vi "LED Main.vi"   [LabVIEW 2016]
uses:
  GlobalVI.vi
  <vilib>/Utility/error.llb/Error Cluster From Error Code.vi
  <vilib>/rvi/errors/niLvFpgaAdjustHostInterfaceError.vi
  <vilib>/rvi/interface/nirviMethod/nirviMethod.xnode
  <vilib>/FPGAPlugInAG/Dynamic/niLvFpga_WriteFifo_Dynamic.vi
  <vilib>/rvi/errors/niLvFpgaMergeErrorWithErrorCode.vi
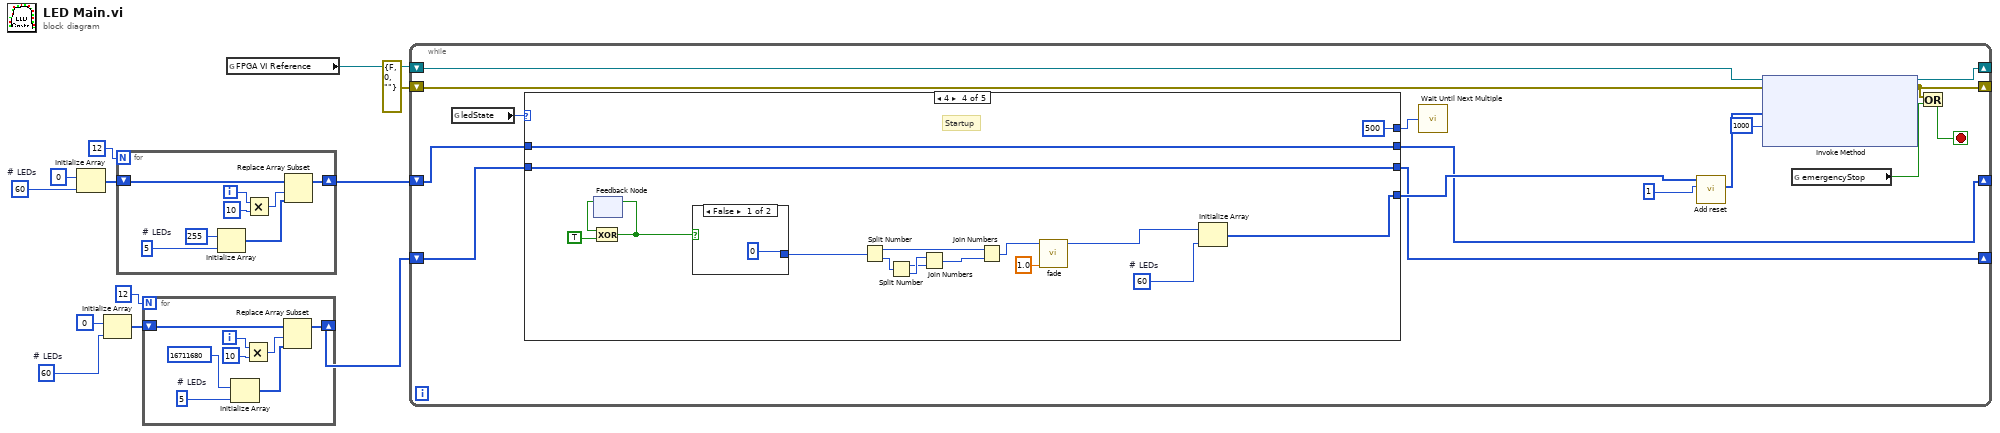
[diagram p0: block diagram]
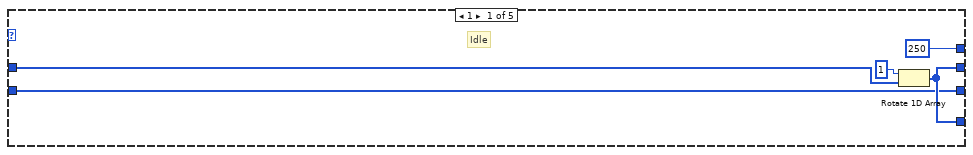
[diagram p2: hidden frame]
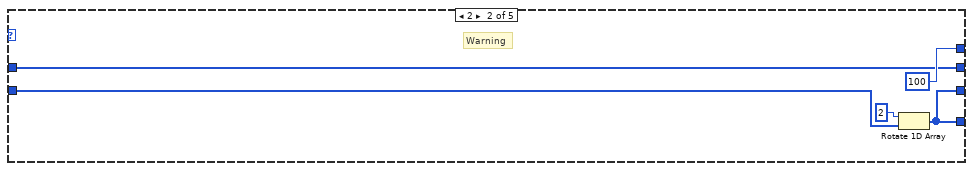
[diagram p3: hidden frame]
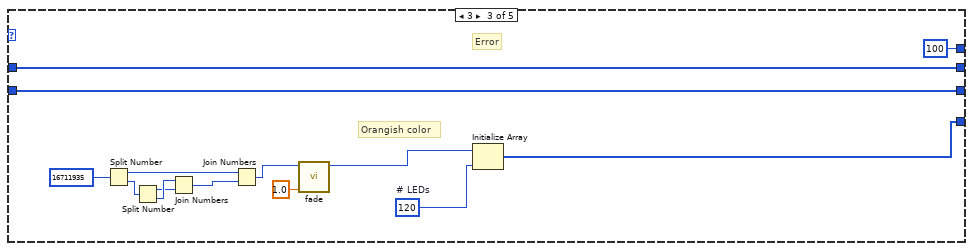
[diagram p4: hidden frame]
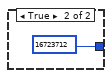
[diagram p5: hidden frame]
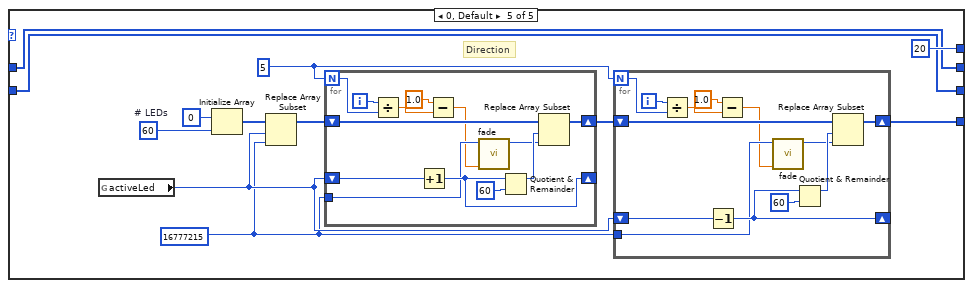
[diagram p6: hidden frame]
diagram:
  w7 = 60  # # LEDs
  w11 = 60  # # LEDs
  n1 = Initialize Array(u32 0 ("Color"), w11) -> (w9:u32[])
  n2 = Initialize Array(u32 0 ("Color"), w7) -> (w5:u32[])
  n3 = for {
    N: 12 -> [_]
    shift-right: [w19] -> w4
    shift-left: w9 -> [w20]
    i -> [w15]
    w18 = 5  # # LEDs
    n4 = Initialize Array(u32 255 ("Color"), w18) -> (w16:u32[])
    n5 = Multiply(x=w15, y=10) -> (x*y=w13:i32)
    n6 = Replace Array Subset(array=w20, new element=w16, index=w13) -> (w19:u32[])
  }
  n7 = for {
    N: 12 -> [_]
    shift-right: [w27] -> w3
    shift-left: w5 -> [w28]
    i -> [w23]
    w26 = 5  # # LEDs
    n8 = Initialize Array(u32 16711680 ("Color"), w26) -> (w24:u32[])
    n9 = Multiply(x=w23, y=10) -> (x*y=w21:i32)
    n10 = Replace Array Subset(array=w28, new element=w24, index=w21) -> (w27:u32[])
  }
  n11 = global read "GlobalVI.vi" "FPGA VI Reference"() -> (w2:refnum<k20>)
  n12 = while {
    shift-right: [w41] -> _
    shift-left: errorcluster {"status"=FALSE, "code"=0, "source"=""} ("error out") -> [w29]
    shift-right: [w44] -> _
    shift-left: w2 -> [w43]
    shift-right: [w32] -> _
    shift-left: w3 -> [w35]
    shift-right: [w33] -> _
    shift-left: w4 -> [w34]
    stop <- w40 stop-if-true
    n13 = global read "GlobalVI.vi" "ledState"() -> (w31:i32)
    n14 = case shown="4" w31 {
      tunnel: [w46 w50 w64 w73 w94] -> w37
      tunnel: [u32 250 ("Count(mSec)") u32 100 ("Count(mSec)") u32 100 ("Count(mSec)") u32 500 ("Count(mSec)") u32 20 ("Count(mSec)")] -> w36
      tunnel: w34 -> [w47 w51 w68 w75 w91]
      tunnel: w35 -> [w45 w52 w65 w74 w92]
      tunnel: [w46 w51 w68 w75 w91] -> w33
      tunnel: [w45 w50 w65 w74 w92] -> w32
      frame 1 {
        # "Idle"
        n15 = Rotate 1D Array(1:w47, 2:1 ("n")) -> (0:w46:u32[])
      }
      frame 2 {
        # "Warning"
        n16 = Rotate 1D Array(1:w52, 2:2 ("n")) -> (0:w50:u32[])
      }
      frame 3 {
        w67 = 120  # # LEDs
        # "Error"
        # "Orangish color"
        n17 = Split Number(x=u32 16711935) -> (hi(x)=w59:u16, lo(x)=w63:u16)
        n18 = Split Number(x=w63) -> (hi(x)=w61:u8, lo(x)=w62:u8)
        n19 = Join Numbers(hi=w62, lo=w61) -> ((hi.lo)=w60:u16)
        n20 = Join Numbers(hi=w59, lo=w60) -> ((hi.lo)=w58:u32)
        n21 = call "fade.vi"("Brightness"=1.0, "In"=w58) -> ("Out"=w57:u32)  [unwired: 9 in]
        n22 = Initialize Array(w57, w67) -> (w64:u32[])
      }
      frame 4 {
        w85 = 60  # # LEDs
        # "Startup"
        n23 = feedback #1() -> (w71:bool)  [unwired: 1 in]
        n24 = Exclusive Or(1:TRUE ("y"), 2:w71) -> (0:w70:bool)
        n25 = feedback-in #1(w70) -> ()
        n26 = case shown="False" w70 {
          tunnel: [u32 0 ("x") u32 16723712 ("x")] -> w69
          frame False {
          }
          frame True {
          }
        }
        n27 = Split Number(x=w69) -> (hi(x)=w80:u16, lo(x)=w84:u16)
        n28 = Split Number(x=w84) -> (hi(x)=w82:u8, lo(x)=w83:u8)
        n29 = Join Numbers(hi=w83, lo=w82) -> ((hi.lo)=w81:u16)
        n30 = Join Numbers(hi=w80, lo=w81) -> ((hi.lo)=w79:u32)
        n31 = call "fade.vi"("Brightness"=1.0, "In"=w79) -> ("Out"=w78:u32)  [unwired: 9 in]
        n32 = Initialize Array(w78, w85) -> (w73:u32[])
      }
      frame 0, Default {
        w88 = 5
        w89 = u32 16777215
        w98 = 60  # # LEDs
        # "Direction"
        n33 = global read "GlobalVI.vi" "activeLed"() -> (w90:i32)
        n34 = Initialize Array(u32 0 ("Color"), w98) -> (w97:u32[])
        n35 = Replace Array Subset(array=w97, new element=w89, index=w90) -> (w96:u32[])
        n36 = for {
          N: w88 -> [w116]
          shift-right: [w124] -> w95
          shift-left: w96 -> [w125]
          shift-right: [w120] -> _
          shift-left: w90 -> [w123]
          tunnel: w89 -> [w119]
          i -> [w117]
          n37 = Divide(x=w117, y=w116) -> (x/y=w115:dbl)
          n38 = Increment(x=w123) -> (x+1=w120:i32)
          n39 = Subtract(x=1.0, y=w115) -> (x-y=w114:dbl)
          n40 = call "fade.vi"("Brightness"=w114, "In"=w119) -> ("Out"=w118:u32)  [unwired: 9 in]
          n41 = Quotient & Remainder(x=w120, y=60) -> (x-y*floor(x/y)=w122:i32)  [unwired: 1 out]
          n42 = Replace Array Subset(array=w125, new element=w118, index=w122) -> (w124:u32[])
        }
        n43 = for {
          N: w88 -> [w103]
          shift-right: [w112] -> w94
          shift-left: w95 -> [w111]
          shift-right: [w108] -> _
          shift-left: w90 -> [w110]
          tunnel: w89 -> [w106]
          i -> [w104]
          n44 = Divide(x=w104, y=w103) -> (x/y=w101:dbl)
          n45 = Decrement(x=w110) -> (x-1=w108:i32)
          n46 = Subtract(x=1.0, y=w101) -> (x-y=w102:dbl)
          n47 = call "fade.vi"("Brightness"=w102, "In"=w106) -> ("Out"=w105:u32)  [unwired: 9 in]
          n48 = Quotient & Remainder(x=w108, y=60) -> (x-y*floor(x/y)=w109:i32)  [unwired: 1 out]
          n49 = Replace Array Subset(array=w111, new element=w105, index=w109) -> (w112:u32[])
        }
      }
    }
    n50 = call "Wait Until Next Multiple"("Count(mSec)"=w36) -> ()  [unwired: 1 out]
    n51 = call "Add reset.vi"("x"=u32 1, "Input"=w37) -> ("Output"=w39:u32[])  [unwired: 9 in]
    n52 = xnode "Invoke Method"("FPGA VI Reference In"=w43, "error in"=w29, "Data"=w39, "Timeout (ms)"=1000) -> ("FPGA VI Reference Out"=w44:refnum<k20>, "error out"=w41:errorcluster)  [unwired: 1 out]
    n53 = global read "GlobalVI.vi" "emergencyStop"() -> (w30:bool)
    n54 = Or(x=w41, y=w30) -> (x .or. y?=w40:bool)
  }
